vi "ReleaseLock.vi"(8 "error in (no error)":errorcluster) -> (0 "error out":errorcluster)   [LabVIEW 2019]
uses:
  DataLock.vi
  Global.lvlib
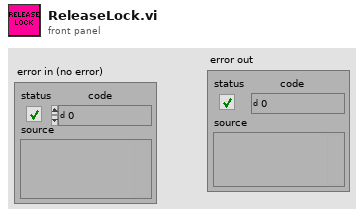
[diagram p1: front panel]
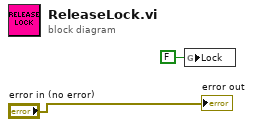
[diagram p0: block diagram]
diagram:
  n1 = global write "DataLock.vi" "Lock"(FALSE ("Lock")) -> ()
  "error out" <- "error in (no error)"
